vi "Clear.vi"(11 "试验项目":T1(ring)) -> ()   [LabVIEW 2012]
uses:
  resultShow.vi
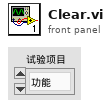
[diagram p1: front panel]
types:
  T1 = enum32{"功能", "输入输出特性", "电流特性", "传感器特性", "空载", "逆向空载", "振动", "7", "8", "9", "10", "11", "12", "13"}
  T2 = enum16{"updatedata", "updatesave", "updateresult", "updateresultempty"}
  T3 = enum16{"selectdata", "selectsave", "selectlist", "selectshow"}
  T4 = cluster{"vaule":dbl, "vaule":dbl, "limitL":dbl, "limitH":dbl}
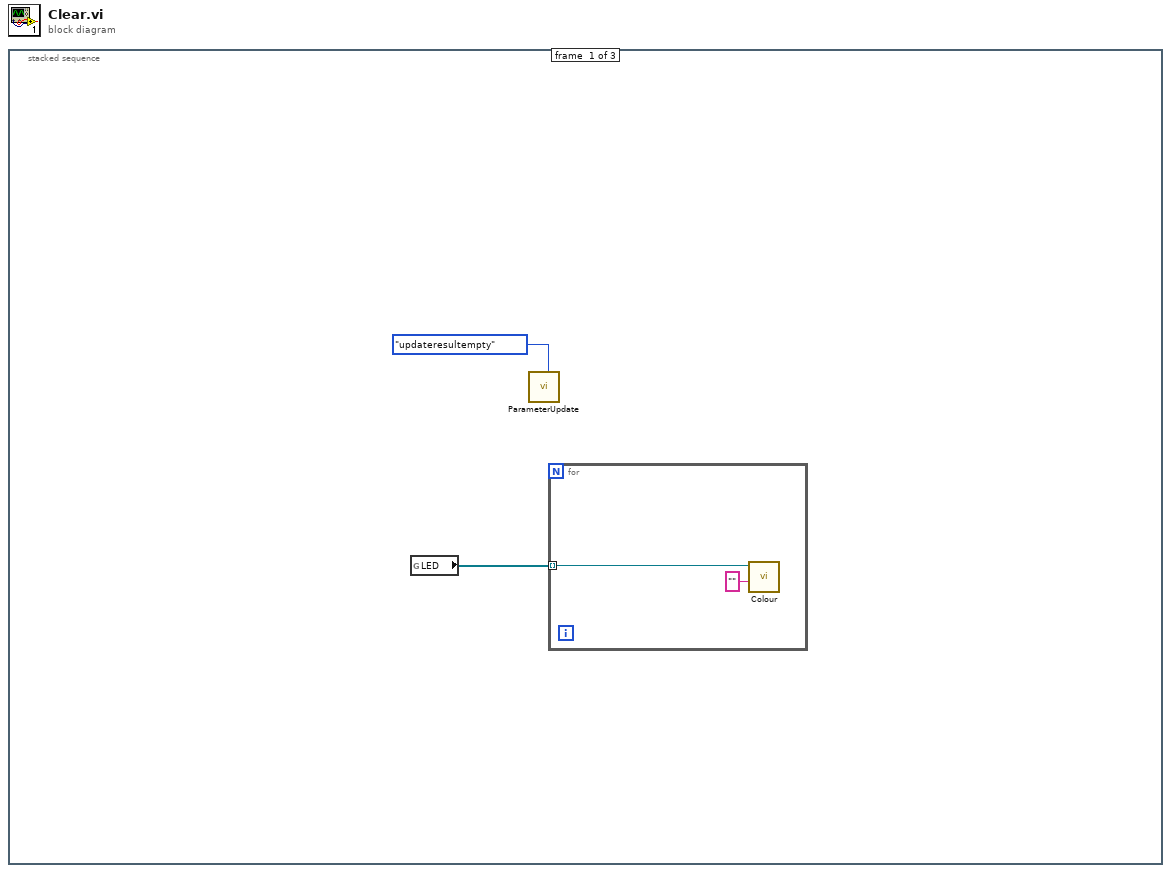
[diagram p0: block diagram]
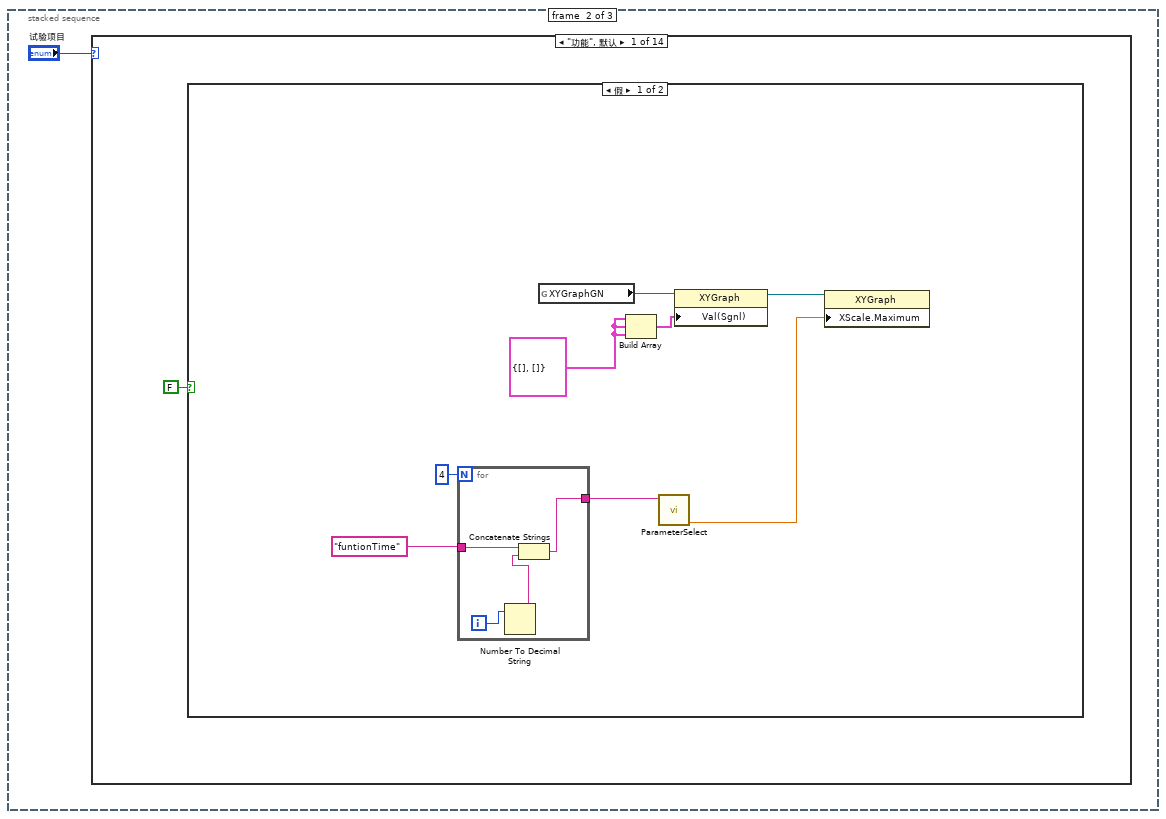
[diagram p2: hidden frame]
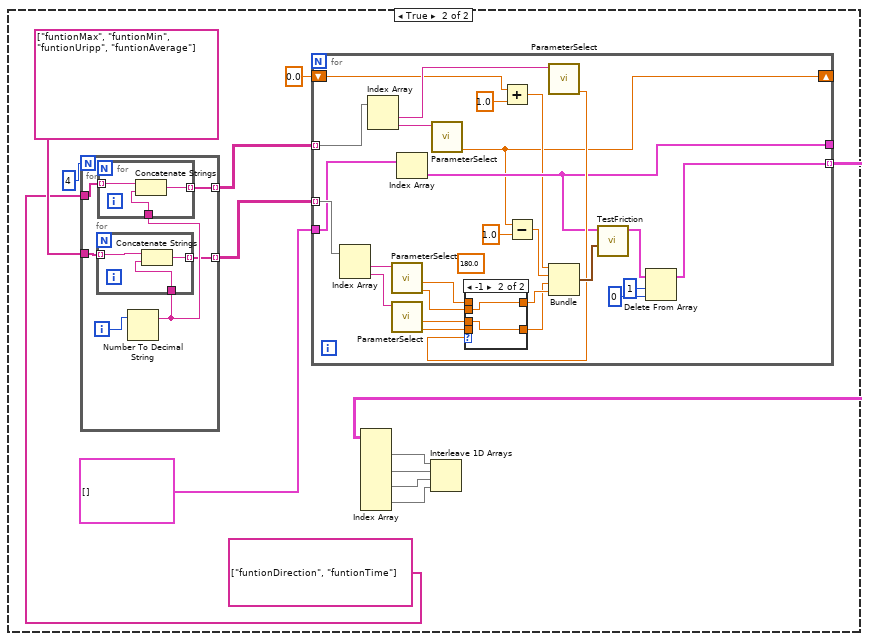
[diagram p3: hidden frame]
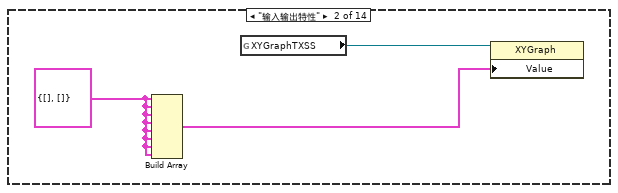
[diagram p5: hidden frame]
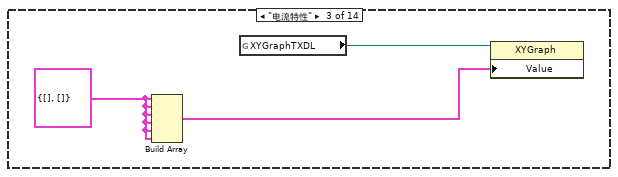
[diagram p6: hidden frame]
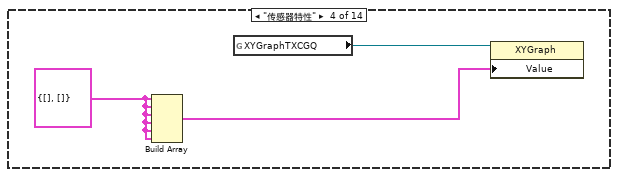
[diagram p7: hidden frame]
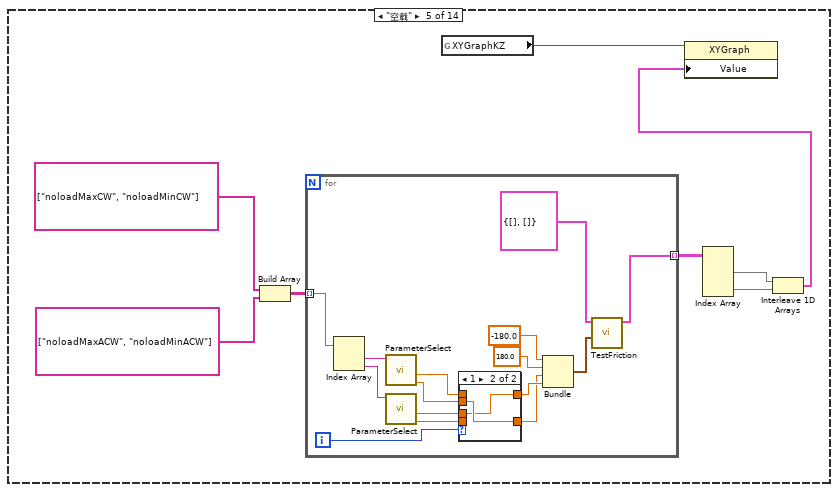
[diagram p8: hidden frame]
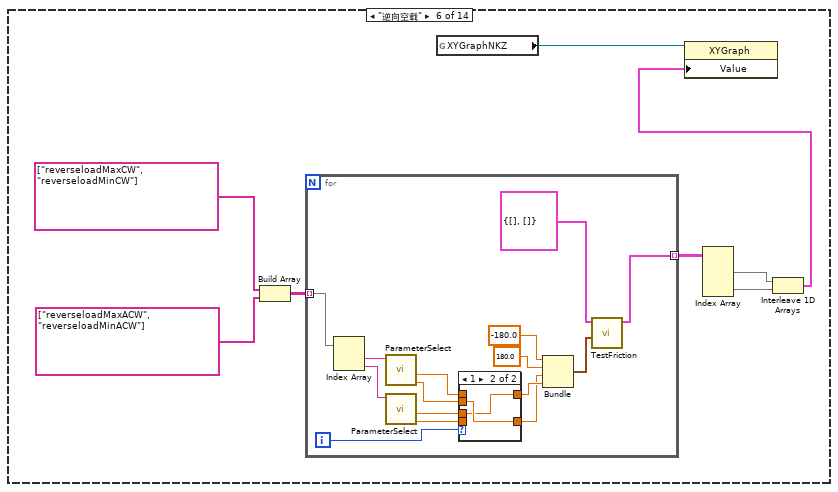
[diagram p10: hidden frame]
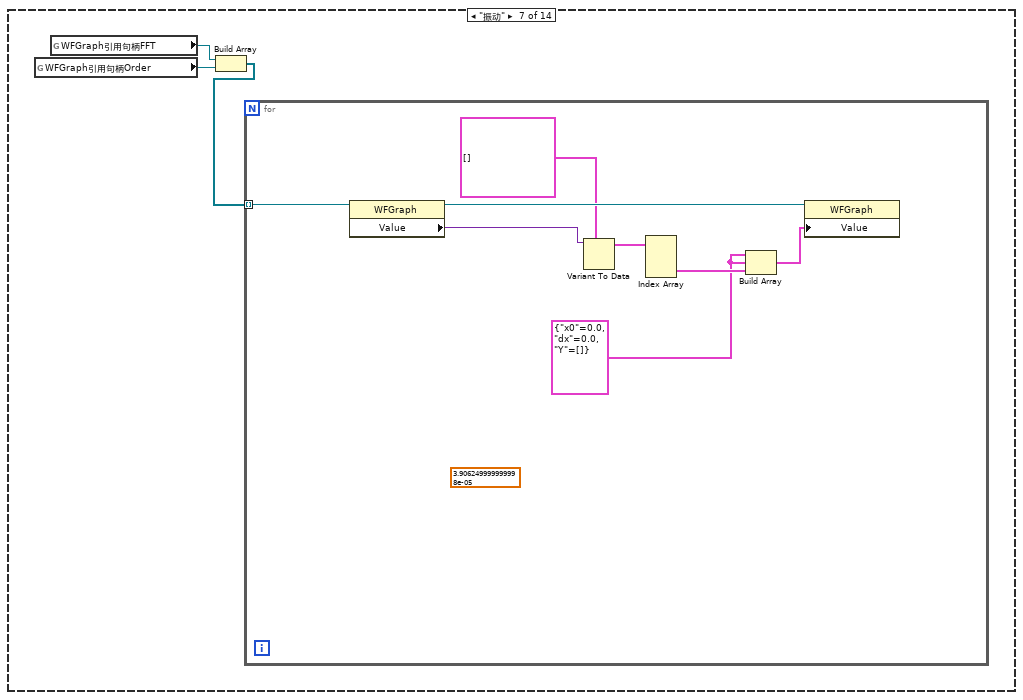
[diagram p12: hidden frame]
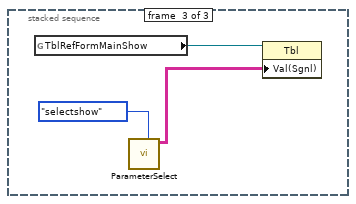
[diagram p20: hidden frame]
diagram:
  n1 = stacked-sequence {
    frame #0 {
      n2 = global read "resultShow.vi" "LED"() -> (w1:refnum<vi>[])
      n3 = call "ParameterUpdate.vi"("模式"=T2."updateresultempty") -> ()  [unwired: 11 in]
      n4 = for {
        tunnel: w1 -> [w4] mode=indexing
        n5 = call "Colour.vi"("result"="", "colourRef"=w4) -> ()  [unwired: 9 in, 1 out]
      }
    }
    frame #1 {
      n6 = case shown="\"功能\", 默认" "试验项目" {
        frame "功能", Default {
          n7 = case shown="假" FALSE {
            frame False {
              w12 = cluster{dbl[], dbl[]} {[], []}
              n8 = for {
                N: 4 -> [_]
                tunnel: "funtionTime" -> [w18]
                tunnel: [w15] -> w9
                i -> [w17]
                n9 = Number To Decimal String(number=w17) -> (decimal integer string=w16:string)  [unwired: 1 in]
                n10 = Concatenate Strings(w18, w16) -> (w15:string)
              }
              n11 = global read "resultShow.vi" "XYGraphGN"() -> (w14:refnum<vi>)
              n12 = Build Array(w12, w12, w12) -> (w13:cluster{dbl[], dbl[]}[])
              n13 = call "ParameterSelect.vi"("parameterName"=w9) -> ("limitL"=w7:dbl)  [unwired: 5 in, 5 out]
              n14 = property class="XYGraph"(reference=w14, "Val(Sgnl)"=w13) -> (reference out=w11:refnum<vi>)  [unwired: 1 in, 1 out]
              n15 = property class="XYGraph"(reference=w11, "XScale.Maximum"=w7) -> ()  [unwired: 1 in, 2 out]
            }
            frame True {
              n16 = for {
                N: 4 -> [_]
                tunnel: string[] ["funtionMax", "funtionMin", "funtionUripp", "funtionAverage"] ("字符串[]") -> [w36]
                tunnel: [w32] -> w27 mode=indexing
                tunnel: [w33] -> w26 mode=indexing
                tunnel: string[] ["funtionDirection", "funtionTime"] ("字符串[]") -> [w31]
                i -> [w35]
                n17 = Number To Decimal String(number=w35) -> (decimal integer string=w34:string)  [unwired: 1 in]
                n18 = for {
                  tunnel: w36 -> [w42] mode=indexing
                  tunnel: w34 -> [w41]
                  tunnel: [w40] -> w32 mode=indexing
                  n19 = Concatenate Strings(w42, w41) -> (w40:string)
                }
                n20 = for {
                  tunnel: w34 -> [w39]
                  tunnel: [w38] -> w33 mode=indexing
                  tunnel: w31 -> [w37] mode=indexing
                  n21 = Concatenate Strings(w37, w39) -> (w38:string)
                }
              }
              n22 = for {
                tunnel: cluster{dbl[], dbl[]}[] [] ("XYData") -> [w58]
                tunnel: w27 -> [w68] mode=indexing
                tunnel: [w50] -> w23 mode=indexing
                tunnel: w26 -> [w57] mode=indexing
                shift-right: [w45] -> _
                shift-left: 0.0 ("limitL") -> [w48]
                tunnel: [w49] -> _
                (unwired) 180.0 ("vaule")
                n23 = Index Array(array=w68) -> (element #1=w67:string, element #2=w66:string)  [unwired: 2 in]
                n24 = Index Array(array=w57) -> (element #1=w55:string, element #2=w56:string)  [unwired: 2 in]
                n25 = call "ParameterSelect.vi"("parameterName"=w67) -> ("limitL"=w60:dbl, "limitH"=w64:dbl)  [unwired: 5 in, 4 out]
                n26 = call "ParameterSelect.vi"("parameterName"=w66) -> ("limitL"=w62:dbl, "limitH"=w59:dbl)  [unwired: 5 in, 4 out]
                n27 = Index Array(array=w58) -> (element=w49:cluster{dbl[], dbl[]})  [unwired: 1 in]
                n28 = call "ParameterSelect.vi"("parameterName"=w56) -> ("limitL"=w45:dbl)  [unwired: 5 in, 5 out]
                n29 = Add(x=w48, y=1.0 ("vaule")) -> (x+y=w47:dbl)
                n30 = Subtract(x=w45, y=1.0 ("vaule")) -> (x-y=w44:dbl)
                n31 = call "ParameterSelect.vi"("parameterName"=w55) -> ("limitL"=w54:dbl)  [unwired: 5 in, 5 out]
                n32 = case shown="-1" w54 {
                  tunnel: w64 -> [w70 _]
                  tunnel: [w70 w72] -> w63
                  tunnel: w62 -> [w69 _]
                  tunnel: [w69 w71] -> w61
                  tunnel: w60 -> [_ w72]
                  tunnel: w59 -> [_ w71]
                  frame 1, Default {
                  }
                  frame -1 {
                  }
                }
                n33 = Bundle(w47, w44, "limitH"=w61, "limitL"=w63) -> (w65:cluster{dbl, dbl, "limitH":dbl, "limitL":dbl})  [unwired: 1 in]
                n34 = call "TestFriction.vi"("边界配置"=w65, "原始曲线"=w49) -> ("曲线数组"=w53:cluster{"X":dbl[], "Y":dbl[]}[])  [unwired: 8 in, 1 out]
                n35 = Delete From Array(array=w53, length=1 ("长度"), index=0 ("索引")) -> (array with subset deleted=w50:cluster{"X":dbl[], "Y":dbl[]}[])  [unwired: 1 out]
              }
              n36 = Index Array(array=w23) -> (element #1=w30:cluster{"X":dbl[], "Y":dbl[]}[], element #2=w21:cluster{"X":dbl[], "Y":dbl[]}[], element #3=w22:cluster{"X":dbl[], "Y":dbl[]}[], element #4=w20:cluster{"X":dbl[], "Y":dbl[]}[])  [unwired: 8 in]
              n37 = Interleave 1D Arrays(w30, w21, w22, w20) -> ()  [unwired: 1 out]
            }
          }
        }
        frame "输入输出特性" {
          w73 = cluster{dbl[], dbl[]} {[], []}
          n38 = Build Array(w73, w73, w73, w73, w73, w73, w73, w73) -> (w74:cluster{dbl[], dbl[]}[])
          n39 = global read "resultShow.vi" "XYGraphTXSS"() -> (w75:refnum<vi>)
          n40 = property class="XYGraph"(reference=w75, "Value"=w74) -> ()  [unwired: 1 in, 2 out]
        }
        frame "电流特性" {
          w78 = cluster{dbl[], dbl[]} {[], []}
          n41 = Build Array(w78, w78, w78, w78, w78, w78) -> (w77:cluster{dbl[], dbl[]}[])
          n42 = global read "resultShow.vi" "XYGraphTXDL"() -> (w76:refnum<vi>)
          n43 = property class="XYGraph"(reference=w76, "Value"=w77) -> ()  [unwired: 1 in, 2 out]
        }
        frame "传感器特性" {
          w79 = cluster{dbl[], dbl[]} {[], []}
          n44 = Build Array(w79, w79, w79, w79, w79, w79) -> (w80:cluster{dbl[], dbl[]}[])
          n45 = global read "resultShow.vi" "XYGraphTXCGQ"() -> (w81:refnum<vi>)
          n46 = property class="XYGraph"(reference=w81, "Value"=w80) -> ()  [unwired: 1 in, 2 out]
        }
        frame "空载" {
          n47 = Build Array(string[] ["noloadMaxCW", "noloadMinCW"] ("字符串[]"), string[] ["noloadMaxACW", "noloadMinACW"] ("字符串[]")) -> (w85:string[][])
          n48 = for {
            tunnel: w85 -> [w104] mode=indexing
            tunnel: [w91] -> w82 mode=indexing
            i -> [w98]
            n49 = Index Array(array=w104) -> (element #1=w103:string, element #2=w102:string)  [unwired: 2 in]
            n50 = call "ParameterSelect.vi"("parameterName"=w103) -> ("limitL"=w93:dbl, "limitH"=w97:dbl)  [unwired: 5 in, 4 out]
            n51 = call "ParameterSelect.vi"("parameterName"=w102) -> ("limitL"=w95:dbl, "limitH"=w92:dbl)  [unwired: 5 in, 4 out]
            n52 = case shown="1" w98 {
              tunnel: w97 -> [w106 _]
              tunnel: [w106 w107] -> w96
              tunnel: w95 -> [w105 _]
              tunnel: [w105 w108] -> w94
              tunnel: w93 -> [_ w108]
              tunnel: w92 -> [_ w107]
              frame 0, Default {
              }
              frame 1 {
              }
            }
            n53 = Bundle("vaule"=-180.0, "vaule"=180.0, "limitL"=w94, "limitH"=w96) -> (w101:T4)  [unwired: 1 in]
            n54 = call "TestFriction.vi"("边界配置"=w101, "原始曲线"=cluster{dbl[], dbl[]} {[], []}) -> ("曲线数组"=w91:cluster{"X":dbl[], "Y":dbl[]}[])  [unwired: 8 in, 1 out]
          }
          n55 = global read "resultShow.vi" "XYGraphKZ"() -> (w89:refnum<vi>)
          n56 = Index Array(array=w82) -> (element #1=w84:cluster{"X":dbl[], "Y":dbl[]}[], element #2=w83:cluster{"X":dbl[], "Y":dbl[]}[])  [unwired: 4 in]
          n57 = Interleave 1D Arrays(w84, w83) -> (w88:cluster{"X":dbl[], "Y":dbl[]}[])
          n58 = property class="XYGraph"(reference=w89, "Value"=w88) -> ()  [unwired: 1 in, 2 out]
        }
        frame "逆向空载" {
          n59 = Build Array(string[] ["reverseloadMaxCW", "reverseloadMinCW"] ("字符串[]"), string[] ["reverseloadMaxACW", "reverseloadMinACW"] ("字符串[]")) -> (w112:string[][])
          n60 = for {
            tunnel: w112 -> [w131] mode=indexing
            tunnel: [w118] -> w109 mode=indexing
            i -> [w125]
            n61 = Index Array(array=w131) -> (element #1=w130:string, element #2=w129:string)  [unwired: 2 in]
            n62 = call "ParameterSelect.vi"("parameterName"=w130) -> ("limitL"=w120:dbl, "limitH"=w124:dbl)  [unwired: 5 in, 4 out]
            n63 = call "ParameterSelect.vi"("parameterName"=w129) -> ("limitL"=w122:dbl, "limitH"=w119:dbl)  [unwired: 5 in, 4 out]
            n64 = case shown="1" w125 {
              tunnel: w124 -> [w133 _]
              tunnel: [w133 w134] -> w123
              tunnel: w122 -> [w132 _]
              tunnel: [w132 w135] -> w121
              tunnel: w120 -> [_ w135]
              tunnel: w119 -> [_ w134]
              frame 0, Default {
              }
              frame 1 {
              }
            }
            n65 = Bundle("vaule"=-180.0, "vaule"=180.0, "limitL"=w121, "limitH"=w123) -> (w128:T4)  [unwired: 1 in]
            n66 = call "TestFriction.vi"("边界配置"=w128, "原始曲线"=cluster{dbl[], dbl[]} {[], []}) -> ("曲线数组"=w118:cluster{"X":dbl[], "Y":dbl[]}[])  [unwired: 8 in, 1 out]
          }
          n67 = global read "resultShow.vi" "XYGraphNKZ"() -> (w116:refnum<vi>)
          n68 = Index Array(array=w109) -> (element #1=w111:cluster{"X":dbl[], "Y":dbl[]}[], element #2=w110:cluster{"X":dbl[], "Y":dbl[]}[])  [unwired: 4 in]
          n69 = Interleave 1D Arrays(w111, w110) -> (w115:cluster{"X":dbl[], "Y":dbl[]}[])
          n70 = property class="XYGraph"(reference=w116, "Value"=w115) -> ()  [unwired: 1 in, 2 out]
        }
        frame "振动" {
          n71 = global read "resultShow.vi" "WFGraph引用句柄Order"() -> (w137:refnum<vi>)
          n72 = global read "resultShow.vi" "WFGraph引用句柄FFT"() -> (w138:refnum<vi>)
          n73 = Build Array(w138, w137) -> (w136:refnum<vi>[])
          n74 = for {
            tunnel: w136 -> [w143] mode=indexing
            (unwired) 3.906249999999998e-05 ("dt")
            w139 = cluster{"x0":dbl, "dx":dbl, "Y":dbl[]} {"x0"=0.0, "dx"=0.0, "Y"=[]} ("元素")
            n75 = property class="WFGraph"(reference=w143) -> (reference out=w146:refnum<vi>, "Value"=w145:variant)  [unwired: 1 in, 1 out]
            n76 = Variant To Data(type=cluster{"x0":dbl, "dx":dbl, "Y":dbl[]}[] [] ("FFT 2"), Variant=w145) -> (data=w142:cluster{"x0":dbl, "dx":dbl, "Y":dbl[]}[])  [unwired: 1 in, 1 out]
            n77 = Index Array(array=w142) -> (element #3=w141:cluster{"x0":dbl, "dx":dbl, "Y":dbl[]})  [unwired: 3 in, 2 out]
            n78 = Build Array(w139, w139, w141) -> (w140:cluster{"x0":dbl, "dx":dbl, "Y":dbl[]}[])
            n79 = property class="WFGraph"(reference=w146, "Value"=w140) -> ()  [unwired: 1 in, 2 out]
          }
        }
        frame "7" {
        }
        frame "8" {
        }
        frame "9" {
        }
        frame "10" {
        }
        frame "11" {
        }
        frame "12" {
        }
        frame "13".. {
        }
      }
    }
    frame #2 {
      n80 = global read "resultShow.vi" "TblRefFormMainShow"() -> (w148:refnum<vi>)
      n81 = call "ParameterSelect.vi"("模式"=T3."selectshow") -> ("dataOutAll"=w147:string[][])  [unwired: 5 in, 5 out]
      n82 = property class="Tbl"(reference=w148, "Val(Sgnl)"=w147) -> ()  [unwired: 1 in, 2 out]
    }
  }
